vi "Filter Test.vi"() -> ()   [LabVIEW 2015]
uses:
  <vilib>/Analysis/3filter.llb/Filter Passband Type.ctl
  <vilib>/Analysis/baseanly.llb/Mean (DBL).vi
  <vilib>/Analysis/3filter.llb/Zero Phase Filter (Cascade, DBL).vi
  <vilib>/Analysis/NI_AALBase.lvlib
panel:
  out "error":i32
  out "Filtered":dbl[](graph)
  in  "low cutoff freq: fl":dbl=0.125 format="%#.3f"
  in  "high cutoff freq: fh":dbl=0.45 format="%#.3f"
  out "Signal":dbl[](graph)
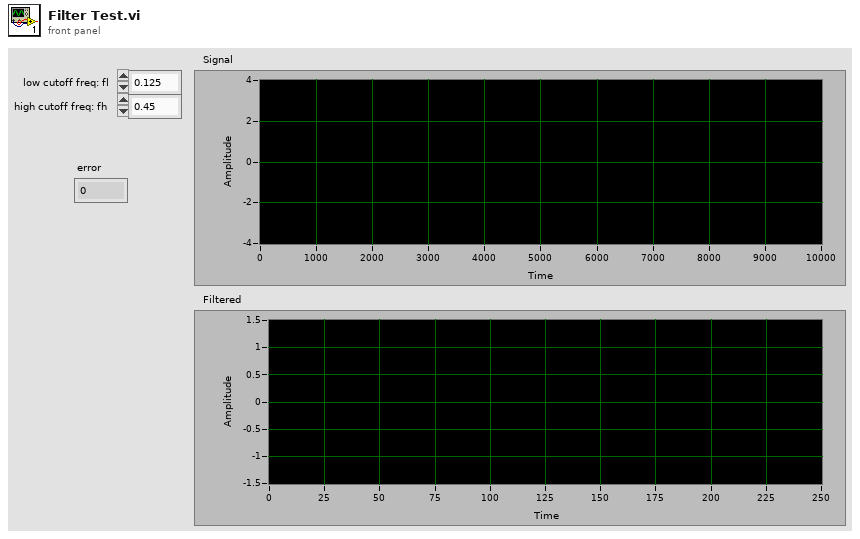
[diagram p1: front panel]
types:
  T1 = typedef "NI_AALBase.lvlib/Filter Passband Type.ctl" = enum32{"Lowpass", "Highpass", "Bandpass", "Bandstop"}
  T2 = cluster{"filter structure":enum32{"IIR 2nd Order", "IIR 4th Order"}, "Reverse Coefficients":dbl[], "Forward Coefficients":dbl[]}
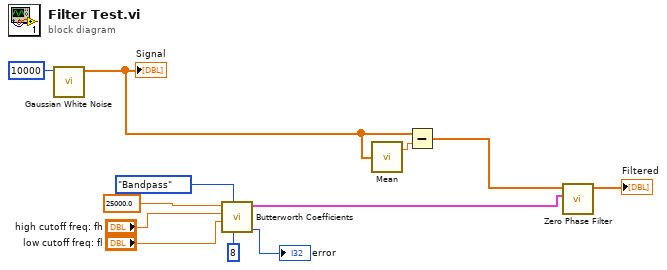
[diagram p0: block diagram]
diagram:
  n1 = call <vilib>:"Gaussian White Noise.vi"("samples"=10000) -> ("Gaussian noise pattern"=w10:dbl[])  [unwired: 9 in, 1 out]
  "Signal" <- w10
  n2 = call <vilib>:"Butterworth Coefficients.vi"("order"=8, "filter type"=Filter_Passband_Type."Bandpass", "low cutoff freq: fl"="low cutoff freq: fl", "high cutoff freq: fh"="high cutoff freq: fh", "sampling freq: fs"=25000.0) -> ("error"=→"error":i32, "IIR Filter Cluster"=w8:T2)  [unwired: 5 in]
  n3 = call-poly <vilib>:"Mean.vi"("X"=w10) -> ("mean"=w11:dbl)  [unwired: 1 out]
  n4 = Subtract(x=w10, y=w11) -> (x-y=w9:dbl[])
  n5 = call-poly <vilib>:"Zero Phase Filter.vi"("IIR Filter Cluster"=w8, "X"=w9) -> ("Filtered X"=→"Filtered":dbl[])  [unwired: 8 in, 1 out]
